vi "TEMPVariant to Attribute.vi"(8 "Error In":errorcluster, 10 "Parameter":variant, 11 "Actor in":refnum<class "Actor.lvclass">) -> (0 "Error Out":errorcluster, 3 "Actor out":refnum<class "Actor.lvclass">)   [LabVIEW 2016, in "AsynchReturn Template.lvclass"]
uses:
  AsynchReturn Template.lvclass
  <vilib>/ActorFramework/Actor/Actor.lvclass
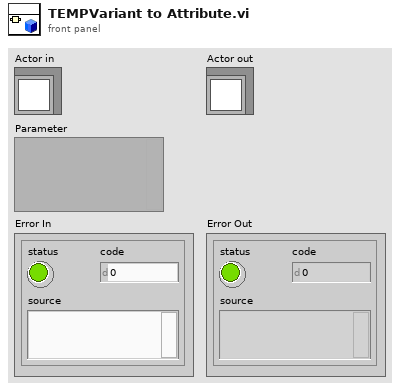
[diagram p1: front panel]
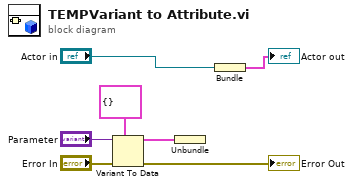
[diagram p0: block diagram]
diagram:
  n1 = Variant To Data(error in="Error In", type=cluster{} {} ("TypeDefCluster"), Variant="Parameter") -> (data=w1:cluster{}, error out=→"Error Out":errorcluster)
  n2 = Unbundle ("Unbundler")(w1) -> ()  [unwired: 1 out]
  n3 = Bundle ("Bundler")(cluster="Actor in") -> (→"Actor out":cluster{void})  [unwired: 1 in]
